vi "Fit VI window to Pane Center.vi"(4 "Error In":errorcluster, 6 "Pane Ref":refnum<vi>, 7 "VI Ref":refnum<vi>) -> (0 "Error Out":errorcluster, 3 "dup VI Ref":refnum<vi>)   [LabVIEW 2017, in "csm-ui-support.lvlib"]
doc: "This VI is designed to center a callee VI's window in a caller VI's window.\n\nAuthored by Brandon Steele\nsupport@mooregoodideas.com\nwww.mooregoodideas.com\n\nCopyright (c) 2010, Moore Good Ideas, Inc.\n\nAll rights reserved.\n\nRedistribution and use in source and binary forms, with or without modification, are permitted provided that the following conditions are met:\n\n * Redistributions of source code must retain the above copyright notice, this list of conditions and the following disclaimer.\n * Redistributions in binary form must reproduce the above copyright notice, this list of conditions and the following disclaimer in the documentation and/or other materials provided with the distribution.\n * Neither the name of Moore Good Ideas, Inc. nor the names of its contributors may be used to endorse or promote products derived from this software without specific prior written permission.\n\nTHIS SOFTWARE IS PROVIDED BY THE COPYRIGHT HOLDERS AND CONTRIBUTORS \"AS IS\" AND ANY EXPRESS OR IMPLIED WARRANTIES, INCLUDING, BUT NOT LIMITED TO, THE IMPLIED WARRANTIES OF MERCHANTABILITY AND FITNESS FOR A PARTICULAR PURPOSE ARE DISCLAIMED. IN NO EVENT SHALL THE COPYRIGHT OWNER OR CONTRIBUTORS BE LIABLE FOR ANY DIRECT, INDIRECT, INCIDENTAL, SPECIAL, EXEMPLARY, OR CONSEQUENTIAL DAMAGES (INCLUDING, BUT NOT LIMITED TO, PROCUREMENT OF SUBSTITUTE GOODS OR SERVICES; LOSS OF USE, DATA, OR PROFITS; OR BUSINESS INTERRUPTION) HOWEVER CAUSED AND ON ANY THEORY OF LIABILITY, WHETHER IN CONTRACT, STRICT LIABILITY, OR TORT (INCLUDING NEGLIGENCE OR OTHERWISE) ARISING IN ANY WAY OUT OF THE USE OF THIS SOFTWARE, EVEN IF ADVISED OF THE POSSIBILITY OF SUCH DAMAGE."
uses:
  csm-ui-support.lvlib
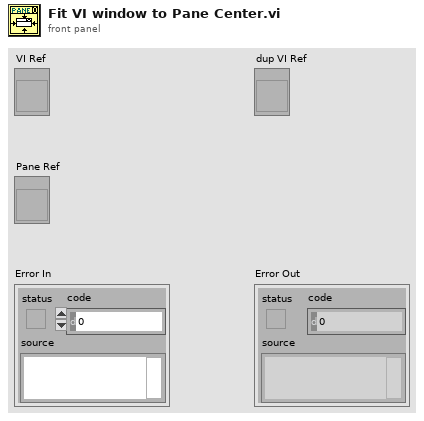
[diagram p1: front panel]
types:
  T1 = typedef "LVRectTypeDef.ctl" = cluster{"Left":i16, "Top":i16, "Right":i16, "Bottom":i16}
  T2 = cluster{"left":i16, "top":i16, "right":i16, "bottom":i16}
  T3 = typedef "LVAllMonitorsDisplayTypeDef.ctl" = cluster{"Bounds":cluster{"Left":i16, "Top":i16, "Right":i16, "Bottom":i16}, "Depth":i16}[]
  T4 = cluster{"Left":i16, "Top":i16, "Right":i16, "Bottom":i16}
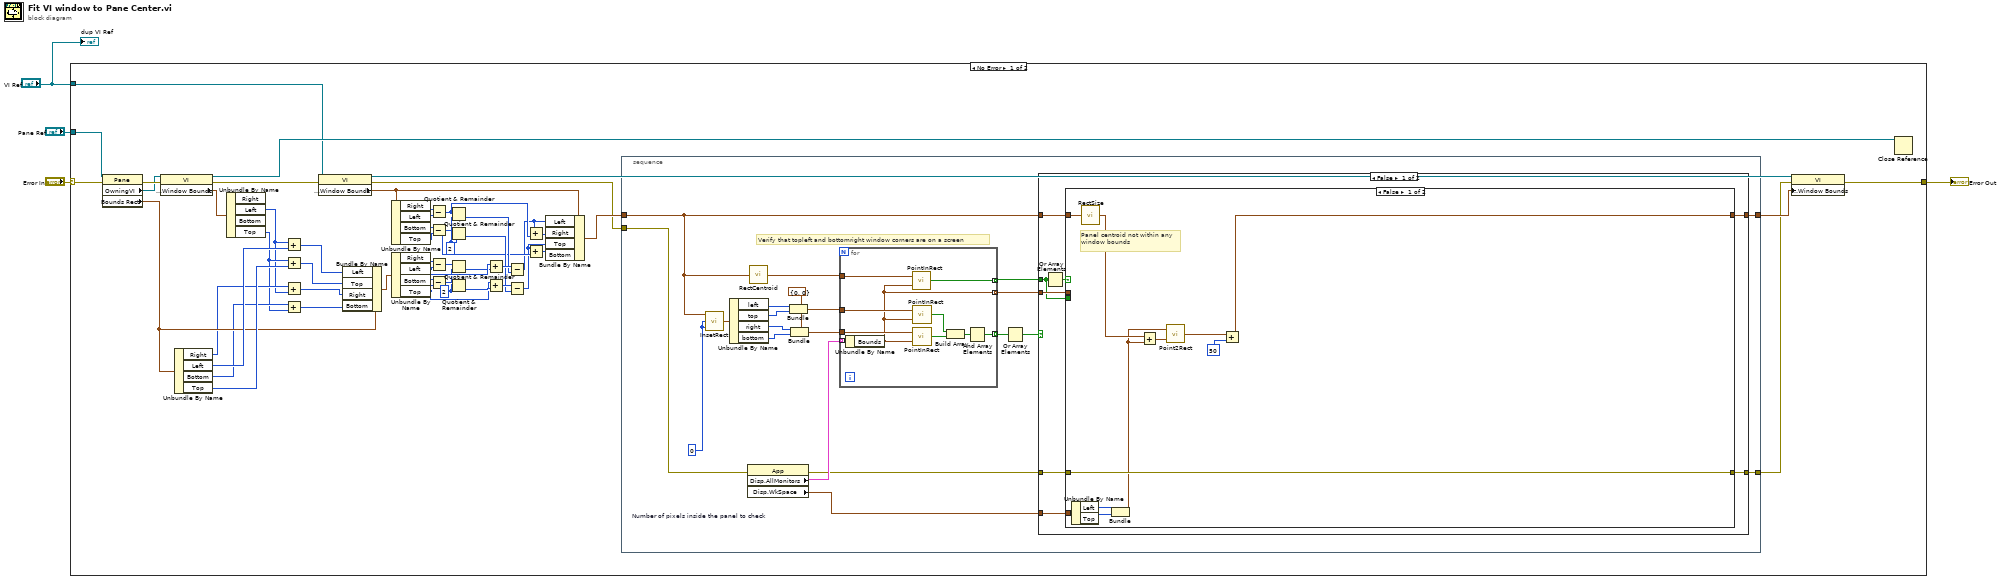
[diagram p0: block diagram]
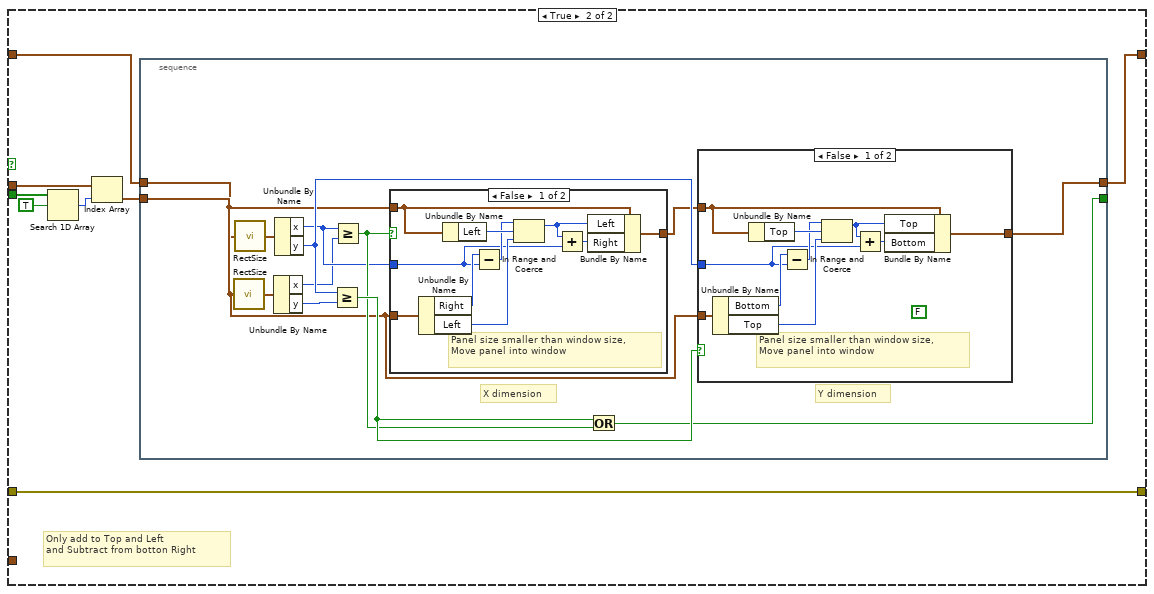
[diagram p2: hidden frame]
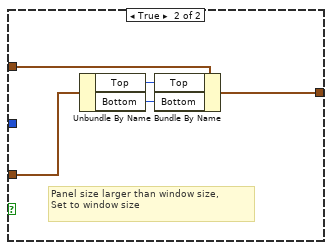
[diagram p3: hidden frame]
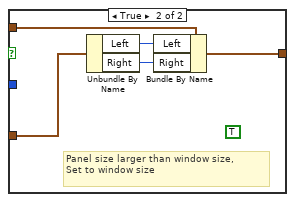
[diagram p4: hidden frame]
diagram:
  n1 = case shown="No Error" "Error In" {
    selector: "Error In" -> [w22 w159]
    tunnel: [w55 w159] -> w4
    tunnel: "Pane Ref" -> [w16 _]
    tunnel: "VI Ref" -> [w5 _]
    frame No Error {
      w49 = i16 2 ("y")
      w33 = i16 2 ("y")
      n2 = property class="Pane"(reference=w16, error in=w22) -> (error out=w21:errorcluster, "OwningVI"=w20:refnum<vi>, "Bounds Rect"=w13:T1)  [unwired: 1 out]
      n3 = property class="VI"(reference=w20, error in=w21) -> (reference out=w32:refnum<vi>, error out=w50:errorcluster, "Front Panel Window:Window Bounds"=w19:T1)
      n4 = Unbundle By Name(w13) -> ("Right"=w10:i16, "Left"=w15:i16, "Bottom"=w9:i16, "Top"=w14:i16)
      n5 = Unbundle By Name(w19) -> ("Left"=w7:i16, "Top"=w8:i16)  [unwired: 2 out]
      n6 = Add(x=w7, y=w15) -> (x+y=w18:i16)
      n7 = Add(x=w8, y=w14) -> (x+y=w17:i16)
      n8 = Add(x=w10, y=w7) -> (x+y=w12:i16)
      n9 = Add(x=w9, y=w8) -> (x+y=w11:i16)
      n10 = property class="VI"(reference=w5, error in=w50) -> (reference out=w36:refnum<vi>, error out=w24:errorcluster, "Front Panel Window:Window Bounds"=w27:T1)
      n11 = Bundle By Name(cluster=w13, "Left"=w18, "Top"=w17, "Right"=w12, "Bottom"=w11) -> (w6:T1)
      n12 = Unbundle By Name(w27) -> ("Right"=w45:i16, "Left"=w46:i16, "Bottom"=w47:i16, "Top"=w48:i16)
      n13 = Unbundle By Name(w6) -> ("Right"=w54:i16, "Left"=w44:i16, "Bottom"=w53:i16, "Top"=w41:i16)
      n14 = Subtract(x=w45, y=w46) -> (x-y=w35:i16)
      n15 = Subtract(x=w47, y=w48) -> (x-y=w34:i16)
      n16 = Subtract(x=w54, y=w44) -> (x-y=w52:i16)
      n17 = Subtract(x=w53, y=w41) -> (x-y=w51:i16)
      n18 = Quotient & Remainder(x=w35, y=w49) -> (floor(x/y)=w39:i16)  [unwired: 1 out]
      n19 = Quotient & Remainder(x=w34, y=w49) -> (floor(x/y)=w37:i16)  [unwired: 1 out]
      n20 = Quotient & Remainder(x=w52, y=w33) -> (floor(x/y)=w43:i16)  [unwired: 1 out]
      n21 = Quotient & Remainder(x=w51, y=w33) -> (floor(x/y)=w42:i16)  [unwired: 1 out]
      n22 = Add(x=w44, y=w43) -> (x+y=w40:i16)
      n23 = Add(x=w41, y=w42) -> (x+y=w38:i16)
      n24 = Subtract(x=w40, y=w39) -> (x-y=w30:i16)
      n25 = Subtract(x=w38, y=w37) -> (x-y=w29:i16)
      n26 = Add(x=w30, y=w35) -> (x+y=w28:i16)
      n27 = Add(x=w29, y=w34) -> (x+y=w31:i16)
      n28 = Bundle By Name(cluster=w27, "Left"=w30, "Right"=w28, "Top"=w29, "Bottom"=w31) -> (w26:T1)
      n29 = stacked-sequence {
        tunnel: [w66] -> w23
        tunnel: [w57] -> w25
        tunnel: w24 -> [w59]
        tunnel: w26 -> [w73]
        frame #0 {
          w68 = i16 0  # Number of pixels inside the panel to check
          w72 = cluster{"x":i16, "y":i16} {"x"=0, "y"=0} ("point")
          # "Verify that topleft and bottomright window corners are on a screen"
          n30 = call <vilib>:"InsetRect.vi"("dv"=w68, "dh"=w68, "rect"=w73) -> ("inset rect"=w62:T2)
          n31 = Unbundle By Name(w62) -> ("left"=w60:i16, "top"=w61:i16, "right"=w69:i16, "bottom"=w70:i16)
          n32 = property class="App"(error in=w59) -> (error out=w56:errorcluster, "Disp.AllMonitors"=w58:T3, "Disp.WkSpace"=w67:T1)  [unwired: 1 in, 1 out]
          n33 = call <vilib>:"RectCentroid.vi"("rect"=w73) -> ("point"=w74:cluster{"x":i16, "y":i16})
          n34 = Bundle(cluster=w72, "x"=w60, "y"=w61) -> (w63:cluster{"x":i16, "y":i16})
          n35 = Bundle(cluster=w72, "x"=w69, "y"=w70) -> (w71:cluster{"x":i16, "y":i16})
          n36 = for {
            tunnel: w58 -> [w158] mode=indexing
            tunnel: w63 -> [w157]
            tunnel: [w153] -> w64 mode=indexing
            tunnel: w71 -> [w152]
            tunnel: w74 -> [w151]
            tunnel: [w150] -> w75 mode=indexing
            tunnel: [w149] -> w76 mode=indexing
            n37 = Unbundle By Name(w158) -> ("Bounds"=w149:T4)
            n38 = call <vilib>:"PointInRect.vi"("rect"=w149, "point"=w151) -> ("pt in rect"=w150:bool)
            n39 = call <vilib>:"PointInRect.vi"("rect"=w149, "point"=w157) -> ("pt in rect"=w156:bool)
            n40 = call <vilib>:"PointInRect.vi"("rect"=w149, "point"=w152) -> ("pt in rect"=w155:bool)
            n41 = Build Array(w156, w155) -> (w154:bool[])
            n42 = And Array Elements(Boolean array=w154) -> (logical AND=w153:bool)
          }
          n43 = Or Array Elements(Boolean array=w64) -> (logical OR=w65:bool)
          n44 = case shown="False" w65 {
            tunnel: w56 -> [w79 w148]
            tunnel: [w78 w148] -> w66
            tunnel: w73 -> [w83 w147]
            tunnel: [w82 w147] -> w57
            tunnel: w67 -> [w84 _]
            tunnel: w75 -> [w77 _]
            tunnel: w76 -> [w80 _]
            frame False {
              n45 = Or Array Elements(Boolean array=w77) -> (logical OR=w81:bool)
              n46 = case shown="False" w81 {
                tunnel: w84 -> [w95 _]
                tunnel: w83 -> [w91 w98]
                tunnel: [w89 w96] -> w82
                tunnel: w80 -> [_ w100]
                tunnel: w79 -> [w88 w103]
                tunnel: [w88 w103] -> w78
                tunnel: w77 -> [_ w102]
                frame False {
                  # "Panel centroid not within any\nwindow bounds"
                  n47 = Unbundle By Name(w95) -> ("Left"=w94:i16, "Top"=w93:i16)
                  n48 = call <vilib>:"RectSize.vi"("rect"=w91) -> ("point"=w87:cluster{"x":i16, "y":i16})
                  n49 = Bundle("Left"=w94, "Top"=w93) -> (w85:cluster{"Left":i16, "Top":i16})  [unwired: 1 in]
                  n50 = Add(x=w87, y=w85) -> (x+y=w86:cluster{i16, i16})
                  n51 = call <vilib>:"Point2Rect.vi"("point b"=w86, "point a"=w85) -> ("rect"=w90:T2)
                  n52 = Add(x=w90, y=i16 50) -> (x+y=w89:T2)
                }
                frame True {
                  # "Only add to Top and Left\nand Subtract from botton Right"
                  n53 = Search 1D Array(1D array=w102, element=TRUE) -> (index of element=w99:i32)  [unwired: 1 in]
                  n54 = Index Array(array=w100, index=w99) -> (element=w97:T4)
                  n55 = stacked-sequence {
                    tunnel: [w104] -> _
                    tunnel: [w114] -> w96
                    tunnel: w97 -> [w113]
                    tunnel: w98 -> [w105]
                    frame #0 {
                      # "X dimension"
                      # "Y dimension"
                      n56 = call <vilib>:"RectSize.vi"("rect"=w113) -> ("point"=w107:cluster{"x":i16, "y":i16})
                      n57 = call <vilib>:"RectSize.vi"("rect"=w105) -> ("point"=w106:cluster{"x":i16, "y":i16})
                      n58 = Unbundle By Name(w107) -> ("x"=w108:i16, "y"=w111:i16)
                      n59 = Unbundle By Name(w106) -> ("x"=w109:i16, "y"=w112:i16)
                      n60 = Greater Or Equal?(x=w112, y=w111) -> (x >= y?=w116:bool)
                      n61 = Greater Or Equal?(x=w109, y=w108) -> (x >= y?=w115:bool)
                      n62 = case shown="False" w115 {
                        tunnel: w113 -> [w141 w142]
                        tunnel: w105 -> [w133 w143]
                        tunnel: w109 -> [w134 _]
                        tunnel: [w132 w144] -> w110
                        frame False {
                          # "Panel size smaller than window size,\nMove panel into window"
                          n63 = Unbundle By Name(w141) -> ("Right"=w137:i16, "Left"=w139:i16)
                          n64 = Unbundle By Name(w133) -> ("Left"=w140:i16)
                          n65 = Subtract(x=w137, y=w134) -> (x-y=w138:i16)
                          n66 = In Range and Coerce(upper limit=w138, x=w140, lower limit=w139) -> (coerced(x)=w136:i16)  [unwired: 1 out]
                          n67 = Add(x=w136, y=w134) -> (x+y=w135:i16)
                          n68 = Bundle By Name(cluster=w133, "Left"=w136, "Right"=w135) -> (w132:T1)
                        }
                        frame True {
                          (unwired) TRUE
                          # "Panel size larger than window size,\nSet to window size"
                          n69 = Unbundle By Name(w142) -> ("Left"=w146:i16, "Right"=w145:i16)
                          n70 = Bundle By Name(cluster=w143, "Left"=w146, "Right"=w145) -> (w144:T1)
                        }
                      }
                      n71 = Or(x=w116, y=w115) -> (x .or. y?=w104:bool)
                      n72 = case shown="False" w116 {
                        tunnel: w113 -> [w126 w131]
                        tunnel: w110 -> [w118 w127]
                        tunnel: w112 -> [w119 _]
                        tunnel: [w117 w128] -> w114
                        frame False {
                          (unwired) FALSE
                          # "Panel size smaller than window size,\nMove panel into window"
                          n73 = Unbundle By Name(w126) -> ("Bottom"=w122:i16, "Top"=w124:i16)
                          n74 = Unbundle By Name(w118) -> ("Top"=w125:i16)
                          n75 = Subtract(x=w122, y=w119) -> (x-y=w123:i16)
                          n76 = In Range and Coerce(upper limit=w123, x=w125, lower limit=w124) -> (coerced(x)=w121:i16)  [unwired: 1 out]
                          n77 = Add(x=w121, y=w119) -> (x+y=w120:i16)
                          n78 = Bundle By Name(cluster=w118, "Top"=w121, "Bottom"=w120) -> (w117:T1)
                        }
                        frame True {
                          # "Panel size larger than window size,\nSet to window size"
                          n79 = Unbundle By Name(w131) -> ("Top"=w130:i16, "Bottom"=w129:i16)
                          n80 = Bundle By Name(cluster=w127, "Top"=w130, "Bottom"=w129) -> (w128:T1)
                        }
                      }
                    }
                  }
                }
              }
            }
            frame True {
            }
          }
        }
      }
      n81 = property class="VI"(reference=w36, error in=w23, "Front Panel Window:Window Bounds"=w25) -> (error out=w55:errorcluster)  [unwired: 1 out]
      n82 = Close Reference(reference=w32) -> ()  [unwired: 1 in, 1 out]
    }
    frame Error {
    }
  }
  "Error Out" <- w4
  "dup VI Ref" <- "VI Ref"
